vi "SO2 43c Serial Data Recording & DECADEv3.6.vi"() -> ()   [LabVIEW 2014]
uses:
  <vilib>/Instr/_visa.llb/VISA Set IO Buffer Mask.ctl
  <vilib>/Platform/TimedLoop/XDataNode/timing_clust.ctl
  <vilib>/Platform/TimedLoop/XDataNode/nitl_modes.ctl
  <vilib>/Platform/TimedLoop/XDataNode/wakeup.ctl
  C:/Program Files (x86)/National Instruments/LabVIEW 2014/examples/Data Communication/Network Streams/Simple Network Streams/support/Network Stream Command.ctl
  <vilib>/Utility/error.llb/whitespace.ctl
  <vilib>/Instr/_visa.llb/VISA Configure Serial Port (Instr).vi
  <vilib>/Utility/tcp.llb/UDP Multicast Write-Only Open.vi
  <vilib>/platform/TimedLoop/XDataNode/XDataNode.xnode
  <vilib>/Platform/TimedLoop/XDataNode/XDNodeRunTimeDep.lvlib
panel:
  out "Default file name":string
  out "Stop File Write":bool
  out "error out 4":errorcluster
  out "Data Array UDP":string[](array[string])
  out "Slope":dbl=0.87463
  out "Offset":dbl
  out "Simulate TWA Conc":dbl
  out "8hr_TWA_limit":i32=490
  out "10mins_STEL_limit":i32=700
  out "Simulate STEL Conc":dbl
  out "Simulate\nconc":bool
  out "q_size 2":i32
  out "8hr_so2_avg 2":dbl=1.0
  out "10min_so2_avg":dbl=1.0
  out "q_size":i32
  in  "Clear Display\nErrors":bool
  in  "dummy2":string="0"
  out "Data Processing":bool
  out "Serial Visa Error":errorcluster
  out "SEPTIC TCP Error Out":errorcluster
  out "TCP packet\nSend to SEPTIC":bool
  in  "Time Stamp\nOffset":u32=1
  out "Data Array TCP":string[](array[string])
  out "UDP packet \nstatus":bool
  out "UDP_Out_Error":errorcluster
  out "FISH TCP Error Out":errorcluster
  out "TCP packet\nSend to FISH":bool
  out "TCP Binary Packet":string
  out "Scan from String Error Counter\nfrom process loop":i32
  out "Read Error Counter\nfrom process loop":i32
  in  "milliseconds to wait":u32=330
  in  "ID":string="«"
  in  "VISA resource name":refnum<visa-resource-name>="ASRL6::INSTR"
  out "Data In Array":string[](array[string])
  out "UDP_ASCII_Out":string
  out "UDP_Pack_num":u32
  out "Flight Number":string
  in  "dummy1":string="00"
  out "Data String":string
  out "Internal packet":string[](array[string])
  out "RAW DATA":string
  in  "stop":bool
  out "Number of Send & Read Error\nfrom Acquire Loop":i32
  out "Command In":string
  # "SO2_conc"
  # "PMT_Volt"
  # "Lamp_Volt"
  # "Lamp_Intensity_Hz"
  # "Internal_Temp_degC"
  # "Reaction_Chamber_Temp_degC"
  # "Reaction_Chamber_Press_mmHg"
  # "Sample_Flow_litre_per_minute"
  # "Flag"
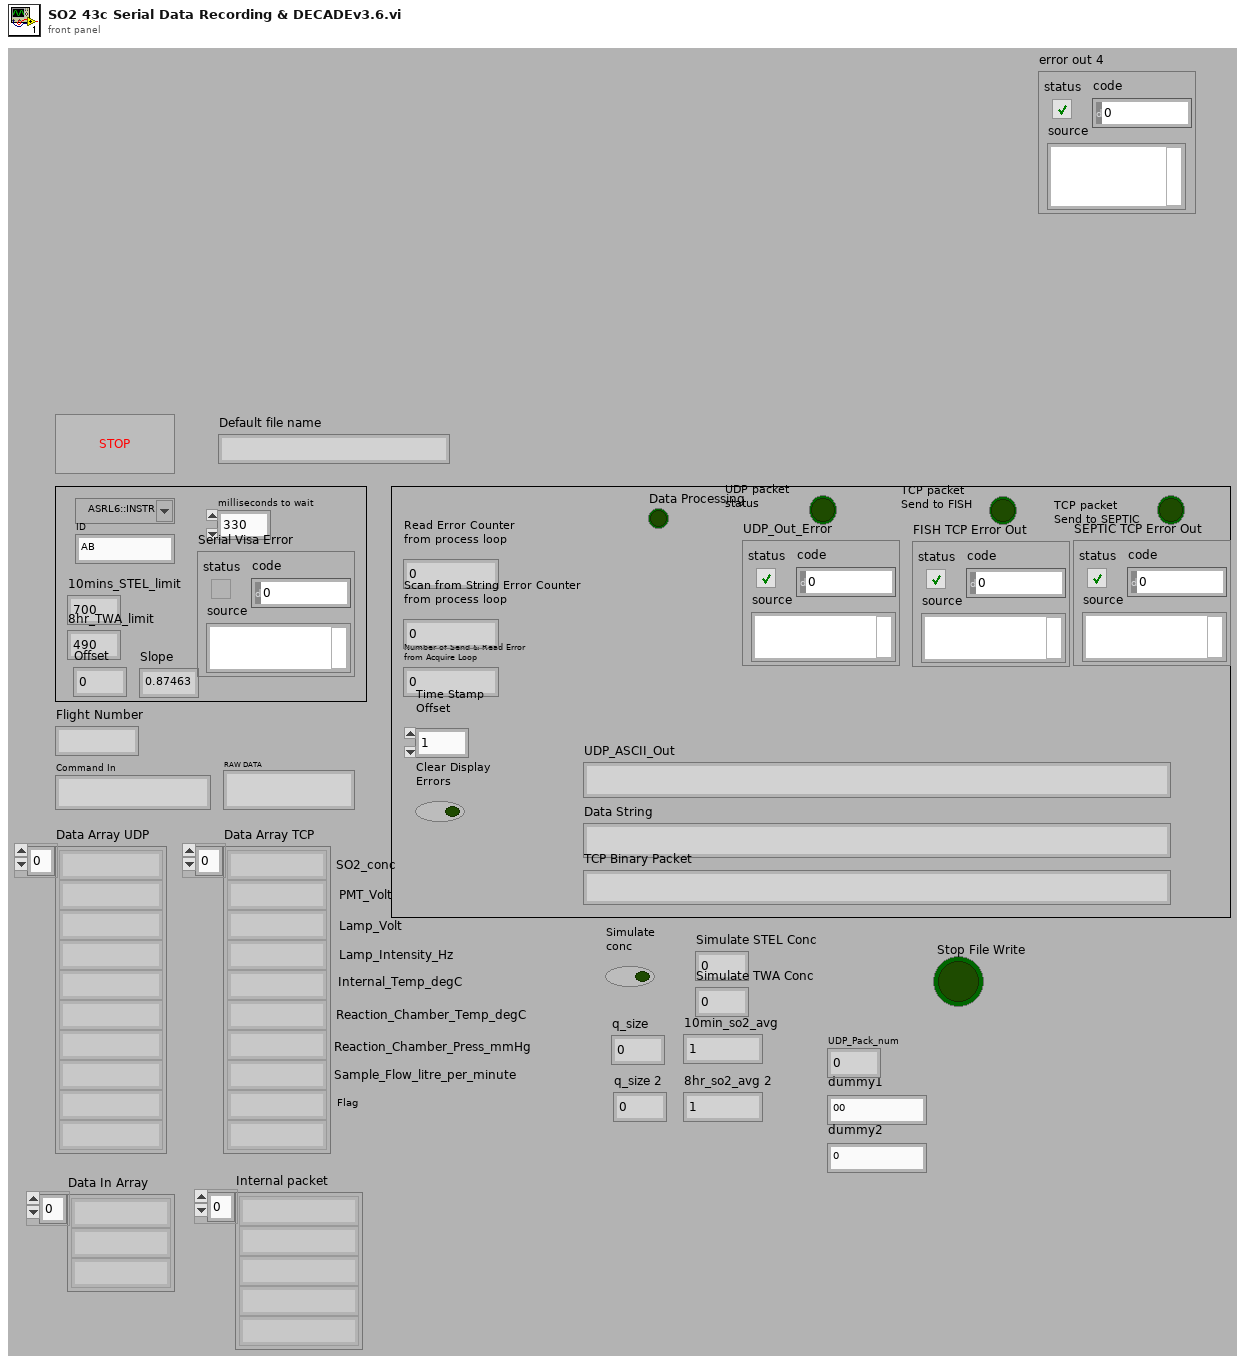
[diagram p1: front panel]
types:
  T1 = typedef "VISA Set IO Buffer Mask.ctl" = u16
  T2 = typedef "Network Stream Command.ctl" = cluster{"Message":string, "Message Data":variant}
  T3 = typedef "XDNodeRunTimeDep.lvlib/timing_clust.ctl" = cluster{"Expected End [f-1]":u64, "Actual End [f-1]":u64, "Finished Late? [f-1]":bool, "Expected End [i-1]":u64, "Actual End [i-1]":u64, "Finished Late? [i-1]":bool, "Expected Start [i]":u64, "Actual Start [i]":u64, "Expected Start [f]":u64, "Actual Start [f]":u64, "Source Name":string, "Structure Name":string, "Period":i64, "Deadline":i64, "Offset":i64, "Start":i64, "Priority":i32, "Timeout":i32, "Mode":T4, "Wakeup Reason":T5, "Error":errorcluster, "Source Type":string, "Secondary Source Type":string, "Global End Time":u64, "Global Start Time":u64, "Frame Duration":u64, "Iteration Duration":u64, "Assigned CPU":i32, "I/O Scan Engine Mode":u32}
  T4 = typedef "XDNodeRunTimeDep.lvlib/nitl_modes.ctl" = enum32{"No Change", "Process missed periods, maintain original phase", "Discard missed periods, maintain original phase", "Process missed periods, ignore original phase", "Discard missed periods, ignore original phase"}
  T5 = typedef "XDNodeRunTimeDep.lvlib/wakeup.ctl" = enum32{"Normal", "Aborted", "Asynchronous wakeup", "Timing source error", "Timed loop error", "Timeout"}
  T6 = enum16{"open", "replace", "create", "open or create", "replace or create", "replace or create with confirmation"}
  T7 = typedef "whitespace.ctl" = u16
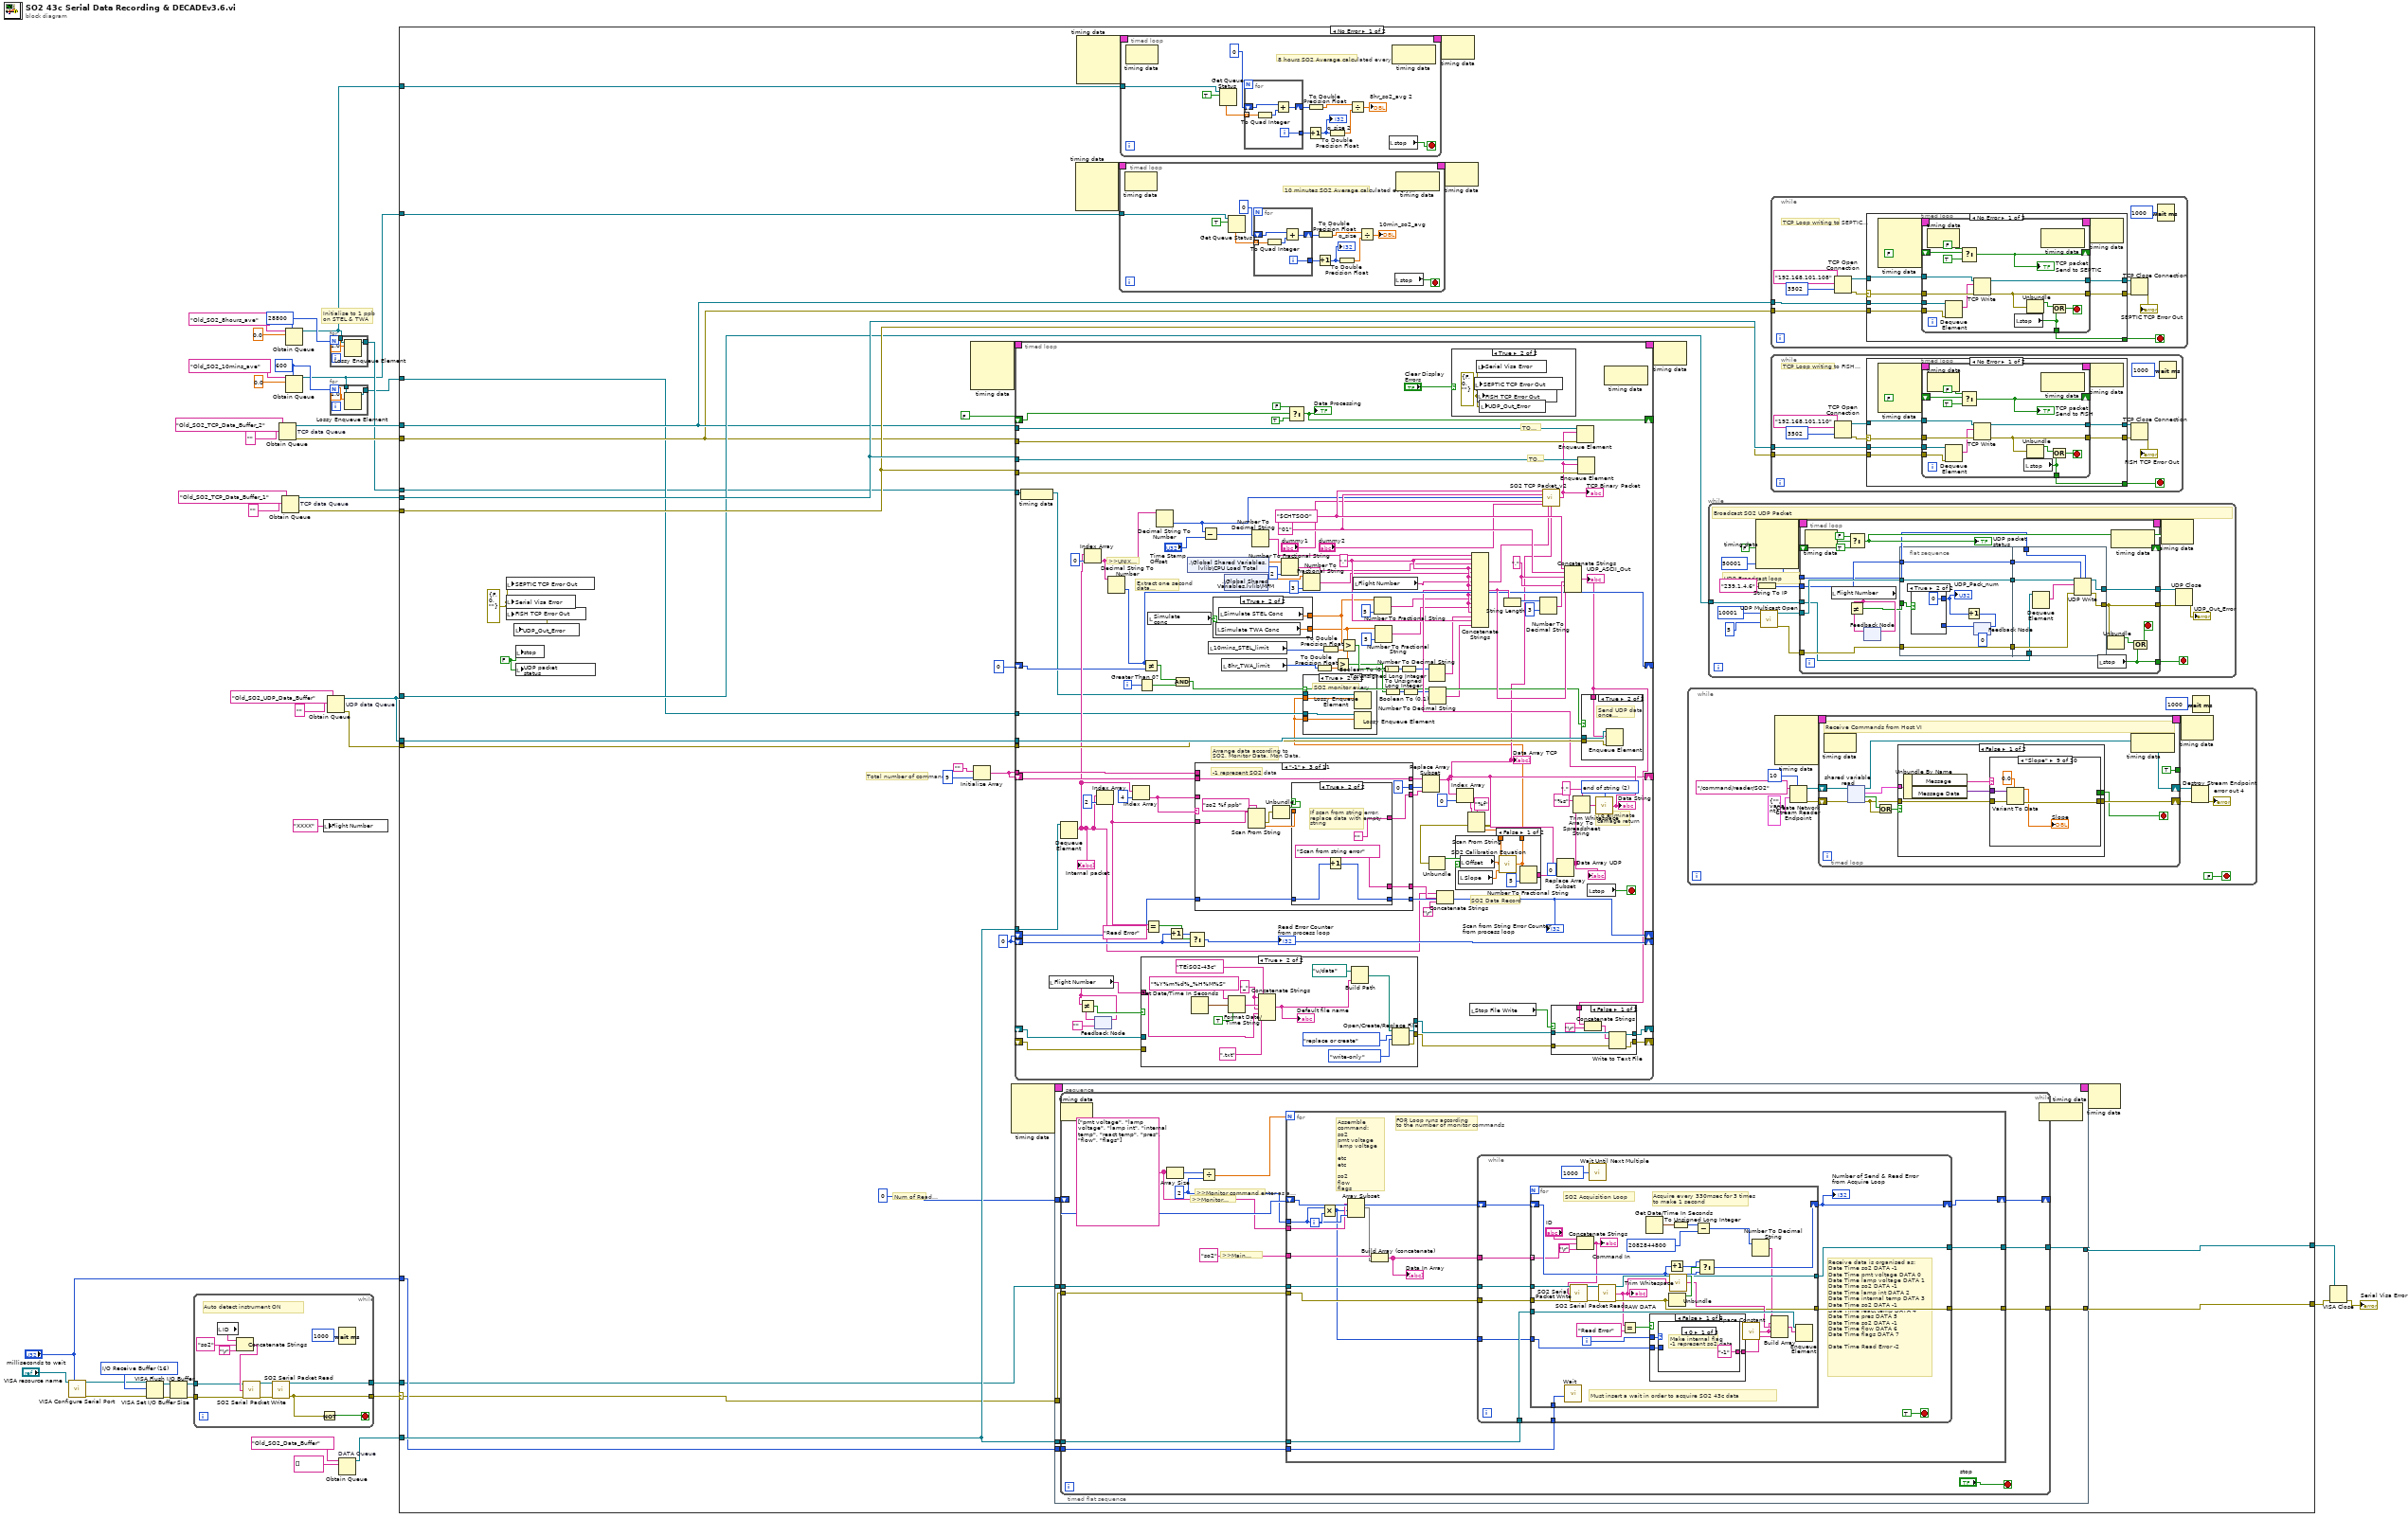
[diagram p0: block diagram]
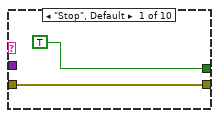
[diagram p2: hidden frame]
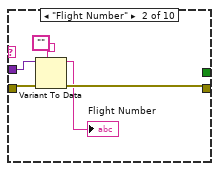
[diagram p3: hidden frame]
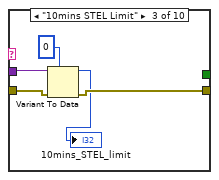
[diagram p4: hidden frame]
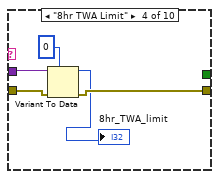
[diagram p5: hidden frame]
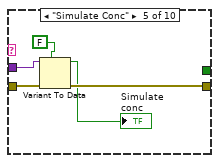
[diagram p6: hidden frame]
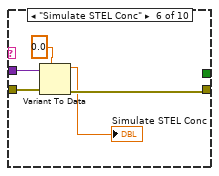
[diagram p7: hidden frame]
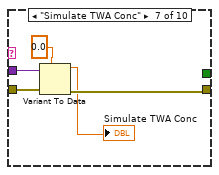
[diagram p8: hidden frame]
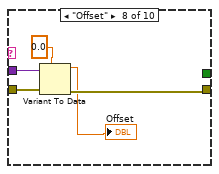
[diagram p9: hidden frame]
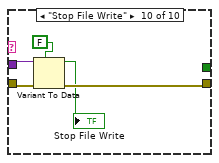
[diagram p10: hidden frame]
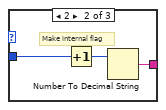
[diagram p12: hidden frame]
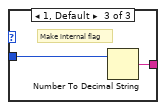
[diagram p13: hidden frame]
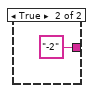
[diagram p14: hidden frame]
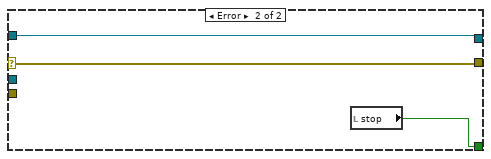
[diagram p15: hidden frame]
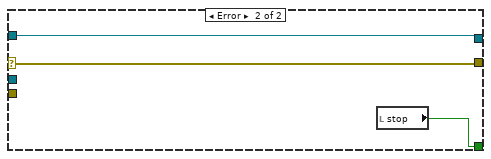
[diagram p17: hidden frame]
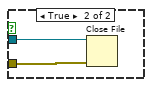
[diagram p19: hidden frame]
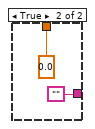
[diagram p20: hidden frame]
diagram:
  w10 = T1 16 items=["I/O Receive Buffer"=16, "I/O Transmit Buffer"=32, "I/O Receive and Transmit Buffer"=48] ("Mask")
  w16 = 28800 ("max queue size (-1, unlimited)")
  w13 = 600 ("max queue size (-1, unlimited)")
  # "Initialise to 1 ppb\non STEL & TWA"
  n1 = call-poly "VISA Configure Serial Port"("VISA resource name"="VISA resource name", "timeout (10sec)"="milliseconds to wait") -> ("VISA resource name out"=w9:refnum<visa-resource-name>, "error out"=w8:errorcluster)  [unwired: 12 in]
  n2 = VISA Set I/O Buffer Size(VISA resource name=w9, mask (16)=w10, error in (no error)=w8) -> (VISA resource name out=w6:refnum<visa-resource-name>, error out=w7:errorcluster)  [unwired: 1 in]
  n3 = VISA Flush I/O Buffer(VISA resource name=w6, error in (no error)=w7) -> (VISA resource name out=w5:refnum<visa-resource-name>, error out=w4:errorcluster)  [unwired: 1 in]
  n4 = while {
    tunnel: w5 -> [w48]
    tunnel: w4 -> [w47]
    tunnel: [w43] -> w3
    tunnel: [w42] -> w2
    stop <- w44 stop-if-true
    # "Auto detect instrument ON"
    n5 = local read "ID"() -> (w51:string)
    n6 = Concatenate Strings(w51, "so2" ("string"), "\r") -> (w49:string)
    n7 = call "SO2 Serial Packet Write.vi"("VISA resource name In"=w48, "Data in"=w49, "error in (no error)"=w47) -> ("VISA resource name Out"=w45:refnum<visa-resource-name>, "error out"=w46:errorcluster)  [unwired: 11 in]
    n8 = call "SO2 Serial Packet Read.vi"("VISA resource In"=w45, "error in"=w46) -> ("VISA resource Out"=w42:refnum<visa-resource-name>, "error out"=w43:errorcluster)  [unwired: 11 in, 1 out]
    n9 = Not(x=w43) -> (.not. x?=w44:bool)
    n10 = Wait (ms)(milliseconds to wait=u32 1000) -> ()  [unwired: 1 out]
  }
  n11 = Obtain Queue "TCP data Queue"(name (unnamed)="Old_SO2_TCP_Data_Buffer_2", element data type="") -> (queue out=w23:refnum<queue>, error out=w22:errorcluster)  [unwired: 3 in, 1 out]
  n12 = Obtain Queue "TCP data Queue"(name (unnamed)="Old_SO2_TCP_Data_Buffer_1", element data type="") -> (queue out=w31:refnum<queue>, error out=w30:errorcluster)  [unwired: 3 in, 1 out]
  n13 = Obtain Queue(max queue size (-1, unlimited)=w16, name (unnamed)="Old_SO2_8hours_ave", element data type=0.0 ("index")) -> (queue out=w15:refnum<queue>)  [unwired: 2 in, 2 out]
  n14 = Obtain Queue(max queue size (-1, unlimited)=w13, name (unnamed)="Old_SO2_10mins_ave", element data type=0.0 ("index")) -> (queue out=w12:refnum<queue>)  [unwired: 2 in, 2 out]
  n15 = local write "Flight Number"("XXXX" ("Flight Number")) -> ()
  n16 = Obtain Queue "UDP data Queue"(name (unnamed)="Old_SO2_UDP_Data_Buffer", element data type="") -> (queue out=w26:refnum<queue>, error out=w27:errorcluster)  [unwired: 3 in, 1 out]
  n17 = for {
    N: w16 -> [_]
    tunnel: w15 -> [w55]
    tunnel: [w54] -> w14
    n18 = Lossy Enqueue Element(queue=w55, element=1.0) -> (queue out=w54:refnum<queue>)  [unwired: 1 in, 3 out]
  }
  n19 = for {
    N: w13 -> [_]
    tunnel: [w58] -> w11
    tunnel: w12 -> [w56]
    n20 = Lossy Enqueue Element(queue=w56, element=1.0) -> (queue out=w58:refnum<queue>)  [unwired: 1 in, 3 out]
  }
  n21 = Obtain Queue "DATA Queue"(name (unnamed)="Old_SO2_Data_Buffer", element data type=string[] []) -> (queue out=w38:refnum<queue>)  [unwired: 3 in, 2 out]
  n22 = case shown="No Error" w3 {
    selector: w3 -> [w61 w818]
    tunnel: [w92 w818] -> w35
    tunnel: [w91 w817] -> w36
    tunnel: w38 -> [w88 _]
    tunnel: w2 -> [w62 w817]
    tunnel: w31 -> [w81 _]
    tunnel: w30 -> [w80 _]
    tunnel: w26 -> [w79 _]
    tunnel: w27 -> [w78 _]
    tunnel: w26 -> [w77 _]
    tunnel: w23 -> [w75 _]
    tunnel: w22 -> [w74 _]
    tunnel: "milliseconds to wait" -> [w73 _]
    tunnel: w12 -> [w70 _]
    tunnel: w15 -> [w69 _]
    tunnel: w11 -> [w68 _]
    tunnel: w14 -> [w67 _]
    frame No Error {
      w71 = errorcluster {"status"=FALSE, "code"=0, "source"=""} ("UDP Error Out")
      w83 = 0
      w82 = FALSE ("stop")
      # "Num of Read Error"
      # "Total number of commands"
      n23 = local write "SEPTIC TCP Error Out"(w71) -> ()
      n24 = local write "Serial Visa Error"(w71) -> ()
      n25 = local write "FISH TCP Error Out"(w71) -> ()
      n26 = local write "UDP_Out_Error"(w71) -> ()
      n27 = local write "stop"(w82) -> ()
      n28 = local write "UDP packet \nstatus"(w82) -> ()
      n29 = node-c288() -> (w90:T3)  [unwired: 4 in]
      n30 = Initialize Array("", 9) -> (w84:string[])
      n31 = node-c288() -> (w60:T3)  [unwired: 4 in]
      n32 = timed-loop {
        timing: w90 -> [_]
        timing-out: [_] -> w89
        tunnel: w88 -> [w564]
        shift-right: [w481] -> _
        shift-left: w84 -> [w554]
        shift-right: [w545] -> _
        shift-left: w83 -> [w542]
        tunnel: w84 -> [w544]
        shift-right: [w540] -> _
        shift-left: w83 -> [w541]
        tunnel: w81 -> [w535]
        tunnel: w80 -> [w534]
        tunnel: w79 -> [w533]
        tunnel: w78 -> [w532]
        shift-right: [w524] -> _
        shift-left: 0 -> [w527]
        tunnel: w75 -> [w523]
        tunnel: w74 -> [w522]
        shift-right: [w513] -> _
        shift-left: FALSE -> [w516]
        tunnel: w68 -> [w507]
        tunnel: w67 -> [w506]
        shift-right: [w466] -> _
        shift-left: _ -> [w463]
        shift-right: [w465] -> _
        shift-left: _ -> [w461]
        i -> [w525]
        stop <- w562 stop-if-true
        w550 = T7 2 items=["both", "start of string", "end of string"] ("location (both)")
        w505 = ","
        w537 = "01"
        w556 = ","
        w538 = "$CHTSOO"
        # "TO SEPTIC"
        # "TO FISH"
        # "Extract one second data\nfor UDP sending"
        # "Arrange data according to\nSO2, Monitor Data, Mon Data,"
        # "To eliminate\ncarriage return"
        # ">>UNIX TIME>>"
        # "SO2 Data Record"
        n33 = node-c288() -> ()  [unwired: 1 in]
        n34 = local read "Flight Number"() -> (w462:string)
        n35 = Dequeue Element(queue=w564) -> (element=w530:string[])  [unwired: 2 in, 3 out]
        "Internal packet" <- w530
        n36 = Index Array(array=w530, index=0) -> (element=w529:string)
        n37 = feedback #1("" ("Flight Number")) -> (w471:string)
        n38 = Not Equal?(x=w462, y=w471) -> (x != y?=w469:bool)
        n39 = feedback-in #1(w462) -> ()
        n40 = Index Array(array=w530, index=2) -> (element=w548:string)
        n41 = Decimal String To Number(string=w529) -> (number=w524:i32)  [unwired: 2 in, 1 out]
        n42 = Index Array(array=w530, index=4) -> (element=w512:string)
        n43 = Greater Than 0?(x=w525) -> (x > 0?=w528:bool)
        n44 = case shown="True" w469 {
          tunnel: [w566 w569] -> w468
          tunnel: [w565 w568] -> w464
          tunnel: w463 -> [w566 _]
          tunnel: w461 -> [w565 _]
          tunnel: w462 -> [_ w567]
          frame False {
          }
          frame True {
            w576 = "_" ("string")
            n45 = Get Date/Time In Seconds() -> (seconds since 1Jan1904=w577:timestamp)
            n46 = Format Date/Time String(time format string (%c)="%Y%m%d%_%H%M%S", seconds (now)=w577, UTC format=TRUE) -> (date/time string=w580:string)
            n47 = Concatenate Strings("TEiSO2-43c" ("string"), w576, w580, w576, w567, ".txt" ("string")) -> (w574:string)
            "Default file name" <- w574
            n48 = Build Path(base path=path "u:/data", name or relative path=w574) -> (appended path=w570:path)
            n49 = Open/Create/Replace File(file path (use dialog)=w570, operation (0:open)=T6."replace or create", access (0:read/write)=enum16{"read/write", "read-only", "write-only"}."write-only") -> (refnum out=w569:refnum<file>, error out=w568:errorcluster)  [unwired: 3 in, 1 out]
          }
        }
        n50 = Not Equal?(x=w524, y=w527) -> (x != y?=w526:bool)
        n51 = Equal?(x=w548, y="Read Error") -> (x = y?=w546:bool)
        n52 = local read "Simulate\nconc"() -> (w475:bool)
        n53 = Decimal String To Number(string=w529) -> (number=w519:i32)  [unwired: 2 in, 1 out]
        n54 = Increment(x=w542) -> (x+1=w543:i32)
        n55 = Compound Arithmetic op=AND(w526, w528) -> (w508:bool)
        n56 = shared-variable ".\\Global Shared Variables.lvlib\\CPU Load Total"() -> (w459:dbl)  [unwired: 1 in, 1 out]
        n57 = Select(t=w543, s=w546, f=w542) -> (s? t:f=w545:i32)
        "Read Error Counter\nfrom process loop" <- w545
        n58 = case shown="\"-1\"" w512 {
          tunnel: w512 -> [w616 _ _ w652 w673 w694 w716 w738 w760 w782 w804]
          tunnel: w554 -> [w617 _ w631 w653 w674 w695 w717 w739 w761 w783 w805]
          tunnel: w548 -> [_ _ w628 w648 w669 w691 w713 w735 w757 w779 w801]
          tunnel: [w617 w620 w631 w653 w674 w695 w717 w739 w761 w783 w805] -> w488
          tunnel: [w614 _ 0 ("index") w650 w671 w692 w714 w736 w758 w780 w802] -> w487
          tunnel: [_ _ w627 w647 w668 w690 w712 w734 w756 w778 w796] -> w553
          tunnel: w544 -> [_ w620 _ _ _ _ _ _ _ _ _]
          tunnel: w541 -> [w612 w619 w624 w644 w665 w685 w708 w729 w752 w773 w795]
          tunnel: [w612 w619 w623 w643 w664 w684 w707 w728 w751 w772 w794] -> w540
          tunnel: ["Internal False Flag Detected" "" w622 w642 w663 w683 w706 w727 w750 w771 w793] -> w539
          frame "False", Default {
            n59 = Decimal String To Number(string=w616) -> (number=w613:i32)  [unwired: 2 in, 1 out]
            n60 = Add(x=w613, y=1) -> (x+y=w614:i32)
          }
          frame "-2" {
            # "Read Error Detected\nMake all data as a space"
          }
          frame "-1" {
            # "-1 represent SO2 data"
            n61 = Scan From String(format string="so2 %f ppb", input string=w628) -> (error out=w626:errorcluster, output 1=w621:dbl)  [unwired: 3 in, 2 out]
            n62 = Unbundle(w626) -> ("status"=w625:bool)  [unwired: 2 out]
            n63 = case shown="True" w625 {
              tunnel: w621 -> [w632 _]
              tunnel: [w636 ""] -> w627
              tunnel: w624 -> [w635 w640]
              tunnel: [w635 w639] -> w623
              tunnel: ["" "Scan from string error"] -> w622
              frame False {
                # "Extract the concentration\nvalue & fixed format"
                n64 = Number To Fractional String(number=w632, precision (6)=i16 5) -> (F-format string=w636:string)  [unwired: 2 in]
              }
              frame True {
                # "If scan from string error,\nreplace data with empty\nstring"
                n65 = Increment(x=w640) -> (x+1=w639:i32)
              }
            }
          }
          frame "0" {
            # "0 represents pmt voltage -0510 volts"
            n66 = Scan From String(format string="pmt voltage %d volts", input string=w648) -> (error out=w646:errorcluster, output 1=w641:i32)  [unwired: 3 in, 2 out]
            n67 = Decimal String To Number(string=w652) -> (number=w651:i32)  [unwired: 2 in, 1 out]
            n68 = Unbundle(w646) -> ("status"=w645:bool)  [unwired: 2 out]
            n69 = case shown="False" w645 {
              tunnel: w641 -> [w657 _]
              tunnel: [w654 w658] -> w647
              tunnel: w644 -> [w656 w661]
              tunnel: [w656 w660] -> w643
              tunnel: ["" "Scan from string error"] -> w642
              tunnel: [w654 w658] -> _
              frame False {
                # "Extract the actual value\n& fixed format"
                n70 = Number To Decimal String(number=w657) -> (decimal integer string=w654:string)  [unwired: 1 in]
              }
              frame True {
                w658 = ""
                # "If scan from string error,\nreplace data with empty\nstring"
                n71 = Increment(x=w661) -> (x+1=w660:i32)
              }
            }
            n72 = Increment(x=w651) -> (x+1=w650:i32)
          }
          frame "1" {
            # "1 represents lamp voltage; lamp voltage 810 volts"
            n73 = Scan From String(format string="lamp voltage %d volts", input string=w669) -> (error out=w667:errorcluster, output 1=w662:i32)  [unwired: 3 in, 2 out]
            n74 = Decimal String To Number(string=w673) -> (number=w672:i32)  [unwired: 2 in, 1 out]
            n75 = Unbundle(w667) -> ("status"=w666:bool)  [unwired: 2 out]
            n76 = case shown="True" w666 {
              tunnel: w662 -> [w678 _]
              tunnel: [w675 w679] -> w668
              tunnel: w665 -> [w677 w682]
              tunnel: [w677 w681] -> w664
              tunnel: ["" "Scan from string error"] -> w663
              tunnel: [w675 w679] -> _
              frame False {
                # "Extract the actual value\n& fixed format"
                n77 = Number To Decimal String(number=w678) -> (decimal integer string=w675:string)  [unwired: 1 in]
              }
              frame True {
                w679 = ""
                # "If scan from string error,\nreplace data with empty\nstring"
                n78 = Increment(x=w682) -> (x+1=w681:i32)
              }
            }
            n79 = Increment(x=w672) -> (x+1=w671:i32)
          }
          frame "2" {
            # "2 represents lamp intensity; lamp int 35867 Hz"
            n80 = Scan From String(format string="lamp int %d Hz", input string=w691) -> (error out=w687:errorcluster, output 1=w688:i32)  [unwired: 3 in, 2 out]
            n81 = Decimal String To Number(string=w694) -> (number=w693:i32)  [unwired: 2 in, 1 out]
            n82 = Unbundle(w687) -> ("status"=w686:bool)  [unwired: 2 out]
            n83 = case shown="True" w686 {
              tunnel: [w696 w701] -> w690
              tunnel: w688 -> [w700 _]
              tunnel: w685 -> [w699 w704]
              tunnel: [w699 w703] -> w684
              tunnel: ["" "Scan from string error"] -> w683
              tunnel: [w696 w701] -> _
              frame False {
                # "Extract the actual value\n& fixed format"
                n84 = Number To Fractional String(number=w700, precision (6)=i16 0) -> (F-format string=w696:string)  [unwired: 2 in]
              }
              frame True {
                w701 = ""
                # "If scan from string error,\nreplace data with empty\nstring"
                n85 = Increment(x=w704) -> (x+1=w703:i32)
              }
            }
            n86 = Increment(x=w693) -> (x+1=w692:i32)
          }
          frame "3" {
            # "3 represents internal temp; internal temp 027.2 deg C, actual 027.2"
            n87 = Scan From String(format string="%[^,], %s %f", input string=w713) -> (error out=w710:errorcluster, output 3=w705:dbl)  [unwired: 7 in, 2 out]
            n88 = Decimal String To Number(string=w716) -> (number=w715:i32)  [unwired: 2 in, 1 out]
            n89 = Unbundle(w710) -> ("status"=w709:bool)  [unwired: 2 out]
            n90 = case shown="True" w709 {
              tunnel: [w718 w723] -> w712
              tunnel: w705 -> [w722 _]
              tunnel: w708 -> [w721 w726]
              tunnel: [w721 w725] -> w707
              tunnel: ["" "Scan from string error"] -> w706
              tunnel: [w718 w723] -> _
              frame False {
                # "Extract the actual value\n& fixed format"
                n91 = Number To Fractional String(number=w722, precision (6)=i16 1) -> (F-format string=w718:string)  [unwired: 2 in]
              }
              frame True {
                w723 = ""
                # "If scan from string error,\nreplace data with empty\nstring"
                n92 = Increment(x=w726) -> (x+1=w725:i32)
              }
            }
            n93 = Increment(x=w715) -> (x+1=w714:i32)
          }
          frame "4" {
            # "4 represents react temp; react temp 045.2 deg C"
            n94 = Scan From String(format string="react temp %f deg C", input string=w735) -> (error out=w731:errorcluster, output 1=w732:dbl)  [unwired: 3 in, 2 out]
            n95 = Decimal String To Number(string=w738) -> (number=w737:i32)  [unwired: 2 in, 1 out]
            n96 = Unbundle(w731) -> ("status"=w730:bool)  [unwired: 2 out]
            n97 = case shown="False" w730 {
              tunnel: [w740 w745] -> w734
              tunnel: w732 -> [w744 _]
              tunnel: w729 -> [w743 w748]
              tunnel: [w743 w747] -> w728
              tunnel: ["" "Scan from string error"] -> w727
              tunnel: [w740 w745] -> _
              frame False {
                # "Extract the actual value\n& fixed format"
                n98 = Number To Fractional String(number=w744, precision (6)=i16 1) -> (F-format string=w740:string)  [unwired: 2 in]
              }
              frame True {
                w745 = ""
                # "If scan from string error,\nreplace data with empty\nstring"
                n99 = Increment(x=w748) -> (x+1=w747:i32)
              }
            }
            n100 = Increment(x=w737) -> (x+1=w736:i32)
          }
          frame "5" {
            # "5 represents chamber pressure; pres 760.0 mm Hg, actual 753.4"
            n101 = Scan From String(format string="%[^,], %s %f", input string=w757) -> (error out=w754:errorcluster, output 3=w749:dbl)  [unwired: 7 in, 2 out]
            n102 = Decimal String To Number(string=w760) -> (number=w759:i32)  [unwired: 2 in, 1 out]
            n103 = Unbundle(w754) -> ("status"=w753:bool)  [unwired: 2 out]
            n104 = case shown="False" w753 {
              tunnel: [w762 w767] -> w756
              tunnel: w749 -> [w766 _]
              tunnel: w752 -> [w765 w770]
              tunnel: [w765 w769] -> w751
              tunnel: ["" "Scan from string error"] -> w750
              tunnel: [w762 w767] -> _
              frame False {
                # "Extract the actual value\n& fixed format"
                n105 = Number To Fractional String(number=w766, precision (6)=i16 1) -> (F-format string=w762:string)  [unwired: 2 in]
              }
              frame True {
                w767 = ""
                # "If scan from string error,\nreplace data with empty\nstring"
                n106 = Increment(x=w770) -> (x+1=w769:i32)
              }
            }
            n107 = Increment(x=w759) -> (x+1=w758:i32)
          }
          frame "6" {
            # "6 represents flow data; flow 0.503 l/m"
            n108 = Scan From String(format string="flow %f l/m", input string=w779) -> (error out=w775:errorcluster, output 1=w776:dbl)  [unwired: 3 in, 2 out]
            n109 = Decimal String To Number(string=w782) -> (number=w781:i32)  [unwired: 2 in, 1 out]
            n110 = Unbundle(w775) -> ("status"=w774:bool)  [unwired: 2 out]
            n111 = case shown="True" w774 {
              tunnel: [w788 ""] -> w778
              tunnel: w776 -> [w787 _]
              tunnel: w773 -> [w786 w791]
              tunnel: [w786 w790] -> w772
              tunnel: ["" "Scan from string error"] -> w771
              frame False {
                # "Extract the actual value\n& fixed format"
                n112 = Number To Fractional String(number=w787, precision (6)=i16 3) -> (F-format string=w788:string)  [unwired: 2 in]
              }
              frame True {
                # "If scan from string error,\nreplace data with empty\nstring"
                n113 = Increment(x=w791) -> (x+1=w790:i32)
              }
            }
            n114 = Increment(x=w781) -> (x+1=w780:i32)
          }
          frame "7" {
            # "7 represents flags data; flags 1c100000"
            n115 = Scan From String(format string="flags %s", input string=w801) -> (error out=w799:errorcluster, output 1=w797:string)  [unwired: 3 in, 2 out]
            n116 = Decimal String To Number(string=w804) -> (number=w803:i32)  [unwired: 2 in, 1 out]
            n117 = Unbundle(w799) -> ("status"=w798:bool)  [unwired: 2 out]
            n118 = case shown="False" w798 {
              tunnel: w797 -> [w808 _]
              tunnel: [w808 ""] -> w796
              tunnel: w795 -> [w807 w811]
              tunnel: [w807 w810] -> w794
              tunnel: ["" "Scan from string error"] -> w793
              frame False {
                # "Extract the actual value\n& fixed format"
              }
              frame True {
                # "If scan from string error,\nreplace data with empty\nstring"
                n119 = Increment(x=w811) -> (x+1=w810:i32)
              }
            }
            n120 = Increment(x=w803) -> (x+1=w802:i32)
          }
        }
        "Scan from String Error Counter\nfrom process loop" <- w540
        n121 = Subtract(x=w519, y="Time Stamp\nOffset") -> (x-y=w520:u32)
        n122 = local read "10mins_STEL_limit"() -> (w473:i32)
        n123 = case shown="True" w475 {
          tunnel: [w600 w602] -> w501
          tunnel: [w599 w601] -> w499
          frame False {
            n124 = local read "10min_so2_avg"() -> (w600:dbl)
            n125 = local read "8hr_so2_avg 2"() -> (w599:dbl)
          }
          frame True {
            n126 = local read "Simulate TWA Conc"() -> (w601:dbl)
            n127 = local read "Simulate STEL Conc"() -> (w602:dbl)
          }
        }
        n128 = local read "8hr_TWA_limit"() -> (w472:i32)
        n129 = shared-variable ".\\Global Shared Variables.lvlib\\MFM"() -> (w457:dbl)  [unwired: 1 in, 1 out]
        n130 = Number To Decimal String(number=w520) -> (decimal integer string=w517:string)  [unwired: 1 in]
        n131 = Number To Fractional String(number=w459, precision (6)=i16 2) -> (F-format string=w455:string)  [unwired: 2 in]
        n132 = Select(t=FALSE, s=w516, f=TRUE) -> (s? t:f=w513:bool)
        "Data Processing" <- w513
        n133 = Number To Fractional String(number=w457, precision (6)=i16 3) -> (F-format string=w454:string)  [unwired: 2 in]
        n134 = To Double Precision Float(number=w472) -> (double precision float=w502:dbl)
        n135 = To Double Precision Float(number=w473) -> (double precision float=w503:dbl)
        n136 = Greater?(x=w499, y=w502) -> (0:w492:bool)
        n137 = Greater?(x=w501, y=w503) -> (0:w494:bool)
        n138 = local read "Flight Number"() -> (w474:string)
        n139 = Number To Fractional String(number=w501, precision (6)=i16 5) -> (F-format string=w498:string)  [unwired: 2 in]
        n140 = Number To Fractional String(number=w499, precision (6)=i16 5) -> (F-format string=w497:string)  [unwired: 2 in]
        n141 = Boolean To (0,1)(Boolean=w494) -> (0, 1=w496:i16)
        n142 = Boolean To (0,1)(Boolean=w492) -> (0, 1=w495:i16)
        n143 = To Unsigned Long Integer(number=w496) -> (unsigned 32bit integer=w490:u32)
        n144 = To Unsigned Long Integer(number=w495) -> (unsigned 32bit integer=w489:u32)
        n145 = Replace Array Subset(array=w488, new element=w553, index=w487) -> (w481:string[])
        "Data Array TCP" <- w481
        n146 = Number To Decimal String(number=w490) -> (decimal integer string=w493:string)  [unwired: 1 in]
        n147 = Number To Decimal String(number=w489) -> (decimal integer string=w491:string)  [unwired: 1 in]
        n148 = Concatenate Strings(w530, w539, "\r") -> ()  [unwired: 1 out]
        n149 = case shown="True" "Clear Display\nErrors" {
          frame False {
          }
          frame True {
            w607 = errorcluster {"status"=FALSE, "code"=0, "source"=""} ("UDP Error Out")
            n150 = local write "SEPTIC TCP Error Out"(w607) -> ()
            n151 = local write "Serial Visa Error"(w607) -> ()
            n152 = local write "FISH TCP Error Out"(w607) -> ()
            n153 = local write "UDP_Out_Error"(w607) -> ()
          }
        }
        n154 = Index Array(array=w481, index=0) -> (element=w485:string)
        n155 = Scan From String(format string="%f", input string=w485) -> (error out=w477:errorcluster, output 1=w483:dbl)  [unwired: 3 in, 2 out]
        n156 = Unbundle(w477) -> ("status"=w476:bool)  [unwired: 2 out]
        n157 = case shown="False" w476 {
          tunnel: w483 -> [w595 _]
          tunnel: [w594 ""] -> w482
          tunnel: [w593 0.0 ("Output")] -> w478
          frame False {
            n158 = local read "Slope"() -> (w591:dbl)
            n159 = local read "Offset"() -> (w592:dbl)
            n160 = call "SO2 Calibration Equation.vi"("Input"=w595, "Offset"=w592, "Slope"=w591) -> ("Output"=w593:dbl)  [unwired: 12 in]
            n161 = Number To Fractional String(number=w593, precision (6)=i16 5) -> (F-format string=w594:string)  [unwired: 2 in]
          }
          frame True {
          }
        }
        n162 = case shown="True" w508 {
          tunnel: w507 -> [_ w606]
          tunnel: w478 -> [_ w603]
          tunnel: w478 -> [_ w605]
          tunnel: w506 -> [_ w604]
          frame False {
          }
          frame True {
            # "SO2 monitor every second"
            n163 = Lossy Enqueue Element(queue=w606, element=w603) -> ()  [unwired: 1 in, 4 out]
            n164 = Lossy Enqueue Element(queue=w604, element=w605) -> ()  [unwired: 1 in, 4 out]
          }
        }
        n165 = local read "Stop File Write"() -> (w467:bool)
        n166 = call "SO2 TCP Packet_v2.vi"("ID"=w538, "Version"=w537, "utc_time"=w519, "dummy1"="dummy1", "dummy2"="dummy2", "Flight Number"=w474, "Data Array"=w481) -> ("TCP Binary Packet"=w521:string)  [unwired: 8 in]
        "TCP Binary Packet" <- w521
        n167 = Replace Array Subset(array=w481, new element=w482, index=0) -> (w480:string[])
        "Data Array UDP" <- w480
        n168 = Array To Spreadsheet String(delimiter (Tab)=",", array=w480, 3:"%s" ("format string")) -> (spreadsheet string=w549:string)
        n169 = Enqueue Element(queue=w523, element=w521, error in (no error)=w522) -> ()  [unwired: 1 in, 3 out]
        n170 = Enqueue Element(queue=w535, element=w521, error in (no error)=w534) -> ()  [unwired: 1 in, 3 out]
        n171 = local read "stop"() -> (w562:bool)
        n172 = call <vilib>:"Trim Whitespace.vi"("string"=w549, "location (both)"=w550) -> ("trimmed string"=w511:string)
        "Data String" <- w511
        n173 = Concatenate Strings(w517, w505, w455, w505, w454, w505, w474, w505, w511, w505, w498, w505, w497, w505, w493, w505, w491) -> (w555:string)
        n174 = String Length(string=w555) -> (length=w559:i32)
        n175 = Number To Decimal String(number=w559, width (-)=i16 3) -> (decimal integer string=w557:string)
        n176 = Concatenate Strings(w538, w537, w556, w557, w556, w555) -> (w460:string)
        "UDP_ASCII_Out" <- w460
        n177 = case shown="False" w467 {
          tunnel: w460 -> [w586 _]
          tunnel: w468 -> [w588 w590]
          tunnel: w464 -> [w587 w589]
          tunnel: [w583 _] -> w466
          tunnel: [w582 _] -> w465
          frame False {
            n178 = Concatenate Strings(w586, "\r") -> (w584:string)
            n179 = Write to Text File(file (use dialog)=w588, text=w584, error in=w587) -> (refnum out=w583:refnum<file>, error out=w582:errorcluster)  [unwired: 2 out]
          }
          frame True {
            n180 = Close File(refnum=w590, error in=w589) -> ()  [unwired: 2 out]
          }
        }
        n181 = case shown="True" w508 {
          tunnel: w533 -> [_ w610]
          tunnel: w532 -> [_ w609]
          tunnel: w460 -> [_ w608]
          frame False {
          }
          frame True {
            # "Send UDP data once\na second"
            n182 = Enqueue Element(queue=w610, element=w608, error in (no error)=w609) -> ()  [unwired: 1 in, 3 out]
          }
        }
        n183 = node-c288() -> ()  [unwired: 1 in, 1 out]
      }
      n184 = timed-sequence {
        timing: w60 -> [_]
        timing-out: [_] -> w59
        tunnel: [w180] -> w92
        tunnel: [w179] -> w91
        tunnel: w88 -> [w178]
        tunnel: 0 -> [w177]
        tunnel: w73 -> [w176]
        tunnel: w62 -> [w175]
        tunnel: w61 -> [w174]
        n185 = timed-flat-sequence {
          tunnel: [w187] -> w180
          tunnel: [w186] -> w179
          tunnel: w178 -> [w185]
          tunnel: w177 -> [w184]
          tunnel: w176 -> [w183]
          tunnel: w175 -> [w182]
          tunnel: w174 -> [w181]
          n186 = node-c288() -> ()  [unwired: 1 in, 1 out]
          n187 = while {
            tunnel: [w190] -> w187
            tunnel: w182 -> [w201]
            tunnel: w181 -> [w200]
            tunnel: [w199] -> w186
            tunnel: w185 -> [w198]
            shift-right: [w196] -> _
            shift-left: w184 -> [w197]
            tunnel: w183 -> [w188]
            stop <- "stop" stop-if-true
            w191 = 2
            w193 = string[] ["pmt voltage", "lamp voltage", "lamp int", "internal temp", "react temp", "pres", "flow", "flags"]
            # ">>Monitor command enter as a pair>>"
            # ">>Main commands>>"
            # ">>Monitor Command>>"
            n188 = Array Size(array=w193) -> (size(s)=w194:i32)
            n189 = Divide(x=w194, y=w191) -> (x/y=w192:dbl)
            n190 = for {
              N: w192 -> [_]
              tunnel: w201 -> [w209]
              tunnel: w200 -> [w208]
              tunnel: [w216] -> w190
              shift-right: [w214] -> w196
              shift-left: w197 -> [w215]
              tunnel: [w213] -> w199
              tunnel: w198 -> [w212]
              tunnel: w193 -> [w205]
              tunnel: "so2" -> [w210]
              tunnel: w191 -> [w206]
              tunnel: w188 -> [w202]
              i -> [w207]
              # "FOR Loop runs according\nto the number of monitor commands"
              # "Assemble command:\nso2\npmt voltage\nlamp voltage\n\netc\netc\n\nso2\nflow\nflags"
              n191 = Multiply(x=w206, y=w207) -> (x*y=w203:i32)
              n192 = Array Subset(array=w205, index=w203, length=w206) -> (w204:string[])
              n193 = Build Array (concatenate)(w210, w204) -> (w211:string[])
              "Data In Array" <- w211
              n194 = while {
                tunnel: [w228] -> w216
                tunnel: w211 -> [w226]
                tunnel: [w224] -> w213
                tunnel: w212 -> [w223]
                tunnel: w208 -> [w222]
                tunnel: w209 -> [w221]
                tunnel: w203 -> [w220]
                shift-right: [w225] -> w214
                shift-left: w215 -> [w227]
                tunnel: w202 -> [w217]
                stop <- TRUE stop-if-true
                # "Receive data is organised as:\nDate Time so2 DATA -1\nDate Time pmt voltage DATA 0\nDate Time lamp voltage DATA 1\nDate Time so2 DATA -1\nDate Time lamp int DATA 2\nDate Time internal temp DATA 3\nDate Time so2 DATA -1\nDate Time react temp DATA 4\nDate Time pres DATA 5\nDate Time so2 DATA -1\nDate Time flow DATA 6\nDate Time flags DATA 7\n\nDate Time Read Error -2"
                n195 = for {
                  tunnel: w222 -> [w245]
                  tunnel: [w246] -> w228
                  tunnel: w226 -> [w243] mode=indexing
                  tunnel: [w247] -> w224
                  tunnel: w223 -> [w253]
                  tunnel: w221 -> [w248]
                  tunnel: w220 -> [w242]
                  shift-right: [w257] -> w225
                  shift-left: w227 -> [w258]
                  tunnel: w217 -> [w231]
                  i -> [w235]
                  # "Must insert a wait in order to acquire SO2 43c data"
                  # "Acquire every 330msec for 3 times\nto make 1 second"
                  # "SO2 Acquisition Loop"
                  n196 = call "Wait"("Count(mSec)"=w231) -> ()  [unwired: 1 out]
                  n197 = Concatenate Strings("ID", w243, "\r") -> (w241:string)
                  "Command In" <- w241
                  n198 = call "SO2 Serial Packet Write.vi"("VISA resource name In"=w248, "Data in"=w241, "error in (no error)"=w245) -> ("VISA resource name Out"=w250:refnum<visa-resource-name>, "error out"=w249:errorcluster)  [unwired: 11 in]
                  n199 = call "SO2 Serial Packet Read.vi"("VISA resource In"=w250, "error in"=w249) -> ("VISA resource Out"=w247:refnum<visa-resource-name>, "Data Out"=w238:string, "error out"=w246:errorcluster)  [unwired: 11 in]
                  "RAW DATA" <- w238
                  n200 = Equal?(x=w238, y="Read Error") -> (x = y?=w236:bool)
                  n201 = Get Date/Time In Seconds() -> (seconds since 1Jan1904=w230:timestamp)
                  n202 = case shown="False" w236 {
                    tunnel: [w261 "-2"] -> w251
                    tunnel: w235 -> [w260 _]
                    tunnel: w242 -> [w259 _]
                    frame False {
                      n203 = case shown="0" w260 {
                        tunnel: ["-1" w265 w267] -> w261
                        tunnel: w259 -> [_ w263 w266]
                        frame 0 {
                          # "Make internal flag\n-1 represent so2 data"
                        }
                        frame 2 {
                          # "Make internal flag"
                          n204 = Increment(x=w263) -> (x+1=w264:i32)
                          n205 = Number To Decimal String(number=w264) -> (decimal integer string=w265:string)  [unwired: 1 in]
                        }
                        frame 1, Default {
                          # "Make internal flag"
                          n206 = Number To Decimal String(number=w266) -> (decimal integer string=w267:string)  [unwired: 1 in]
                        }
                      }
                    }
                    frame True {
                    }
                  }
                  n207 = Increment(x=w258) -> (x+1=w254:i32)
                  n208 = Unbundle(w246) -> ("status"=w255:bool)  [unwired: 2 out]
                  n209 = call <vilib>:"Trim Whitespace.vi"("string"=w238) -> ("trimmed string"=w252:string)  [unwired: 1 in]
                  n210 = To Unsigned Long Integer(number=w230) -> (unsigned 32bit integer=w234:u32)
                  n211 = Subtract(x=w234, y=u32 2082844800) -> (x-y=w229:u32)
                  n212 = Select(t=w254, s=w255, f=w258) -> (s? t:f=w257:i32)
                  n213 = call <vilib>:"Space Constant.vi"() -> ("String"=w239:string)
                  n214 = Number To Decimal String(number=w229) -> (decimal integer string=w232:string)  [unwired: 1 in]
                  n215 = Build Array(w232, w239, w252, w239, w251) -> (w240:string[])
                  n216 = Enqueue Element(queue=w253, element=w240) -> ()  [unwired: 2 in, 3 out]
                }
                "Number of Send & Read Error\nfrom Acquire Loop" <- w225
                n217 = call "Wait Until Next Multiple"("Count(mSec)"=u32 1000) -> ()  [unwired: 1 out]
              }
            }
          }
          n218 = node-c288() -> ()  [unwired: 1 in, 1 out]
        }
      }
      n219 = node-c288() -> (w64:T3)  [unwired: 4 in]
      n220 = node-c288() -> (w66:T3)  [unwired: 4 in]
      n221 = timed-loop {
        tunnel: w70 -> [w282]
        timing: w64 -> [_]
        timing-out: [_] -> w63
        stop <- w283 stop-if-true
        # "10 minutes SO2 Average calculated every second"
        n222 = node-c288() -> ()  [unwired: 1 in, 1 out]
        n223 = Get Queue Status(queue=w282, return elements? (F)=TRUE) -> (elements=w273:dbl[])  [unwired: 1 in, 7 out]
        n224 = for {
          tunnel: w273 -> [w286] mode=indexing
          tunnel: [w290] -> w279
          shift-right: [w289] -> w277
          shift-left: i64 0 -> [w288]
          i -> [w290]
          n225 = To Quad Integer(1:w286) -> (0:w287:i64)
          n226 = Add(x=w288, y=w287) -> (x+y=w289:i64)
        }
        n227 = Increment(x=w279) -> (x+1=w274:i32)
        "q_size" <- w274
        n228 = To Double Precision Float(number=w277) -> (double precision float=w275:dbl)
        n229 = To Double Precision Float(number=w274) -> (double precision float=w276:dbl)
        n230 = Divide(x=w275, y=w276) -> (x/y=→"10min_so2_avg":dbl)
        n231 = local read "stop"() -> (w283:bool)
        n232 = node-c288() -> ()  [unwired: 1 in, 1 out]
      }
      n233 = timed-loop {
        tunnel: w69 -> [w302]
        timing: w66 -> [_]
        timing-out: [_] -> w65
        stop <- w303 stop-if-true
        # "8 hours SO2 Average calculated every second"
        n234 = node-c288() -> ()  [unwired: 1 in, 1 out]
        n235 = Get Queue Status(queue=w302, return elements? (F)=TRUE) -> (elements=w299:dbl[])  [unwired: 1 in, 7 out]
        n236 = for {
          tunnel: w299 -> [w306] mode=indexing
          tunnel: [w310] -> w298
          shift-right: [w309] -> w296
          shift-left: i64 0 -> [w308]
          i -> [w310]
          n237 = To Quad Integer(1:w306) -> (0:w307:i64)
          n238 = Add(x=w308, y=w307) -> (x+y=w309:i64)
        }
        n239 = Increment(x=w298) -> (x+1=w293:i32)
        "q_size 2" <- w293
        n240 = To Double Precision Float(number=w296) -> (double precision float=w294:dbl)
        n241 = To Double Precision Float(number=w293) -> (double precision float=w295:dbl)
        n242 = Divide(x=w294, y=w295) -> (x/y=→"8hr_so2_avg 2":dbl)
        n243 = local read "stop"() -> (w303:bool)
        n244 = node-c288() -> ()  [unwired: 1 in, 1 out]
      }
      n245 = node-c288(w65) -> ()  [unwired: 1 out]
      n246 = node-c288(w63) -> ()  [unwired: 1 out]
      n247 = node-c288(w89) -> ()  [unwired: 1 out]
      n248 = while {
        stop <- FALSE stop-if-true
        n249 = node-c288() -> (w94:T3)  [unwired: 4 in]
        n250 = Create Network Stream Reader Endpoint(7:10 ("reader buffer size"), 9:T2 {"Message"="", "Message Data"=variant} ("Message Cluster"), 11:"/command/reader/SO2" ("reader url")) -> (0:w100:errorcluster, 3:w101:refnum<k21>)  [unwired: 4 in]
        n251 = timed-loop "Host->Target Command Reader" {
          shift-right: [w111] -> w98
          shift-left: w100 -> [w114]
          shift-right: [w112] -> w97
          shift-left: w101 -> [w113]
          tunnel: [TRUE] -> _
          timing: w94 -> [_]
          timing-out: [_] -> w93
          stop <- w105 stop-if-true
          # "Receive Commands from Host VI"
          n252 = node-c288() -> ()  [unwired: 1 in, 1 out]
          n253 = shared-variable-read(w113, w114) -> (w112:refnum<k21>, w107:errorcluster, w109:bool, w110:T2)  [unwired: 1 in]
          n254 = Or(x=w109, y=w107) -> (x .or. y?=w108:bool)
          n255 = case shown="False" w108 {
            selector: w108 -> [_ w170]
            tunnel: w107 -> [w122 w171]
            tunnel: [w121 w171] -> w111
            tunnel: w110 -> [w119 _]
            tunnel: [w120 w170] -> w105
            frame False {
              n256 = Unbundle By Name(w119) -> ("Message"=w118:string, "Message Data"=w117:variant)
              n257 = case shown="\"Slope\"" w118 {
                tunnel: w122 -> [w124 w129 w134 w139 w144 w148 w153 w158 w163 w169]
                tunnel: [w124 w126 w132 w137 w143 w146 w151 w156 w161 w166] -> w121
                tunnel: w117 -> [_ w128 w133 w138 w142 w149 w154 w159 w164 w168]
                tunnel: [TRUE _ _ _ _ _ _ _ _ _] -> w120
                frame "Stop", Default {
                }
                frame "Flight Number" {
                  n258 = Variant To Data(error in=w129, type="", Variant=w128) -> (data=→"Flight Number":string, error out=w126:errorcluster)
                }
                frame "10mins STEL Limit" {
                  n259 = Variant To Data(error in=w134, type=0, Variant=w133) -> (data=→"10mins_STEL_limit":i32, error out=w132:errorcluster)
                }
                frame "8hr TWA Limit" {
                  n260 = Variant To Data(error in=w139, type=0, Variant=w138) -> (data=→"8hr_TWA_limit":i32, error out=w137:errorcluster)
                }
                frame "Simulate Conc" {
                  n261 = Variant To Data(error in=w144, type=FALSE, Variant=w142) -> (data=→"Simulate\nconc":bool, error out=w143:errorcluster)
                }
                frame "Simulate STEL Conc" {
                  n262 = Variant To Data(error in=w148, type=0.0, Variant=w149) -> (data=→"Simulate STEL Conc":dbl, error out=w146:errorcluster)
                }
                frame "Simulate TWA Conc" {
                  n263 = Variant To Data(error in=w153, type=0.0, Variant=w154) -> (data=→"Simulate TWA Conc":dbl, error out=w151:errorcluster)
                }
                frame "Offset" {
                  n264 = Variant To Data(error in=w158, type=0.0, Variant=w159) -> (data=→"Offset":dbl, error out=w156:errorcluster)
                }
                frame "Slope" {
                  n265 = Variant To Data(error in=w163, type=0.0, Variant=w164) -> (data=→"Slope":dbl, error out=w161:errorcluster)
                }
                frame "Stop File Write" {
                  n266 = Variant To Data(error in=w169, type=FALSE, Variant=w168) -> (data=→"Stop File Write":bool, error out=w166:errorcluster)
                }
              }
            }
            frame True {
            }
          }
          n267 = node-c288() -> ()  [unwired: 1 in, 1 out]
        }
        n268 = node-c288(w93) -> ()  [unwired: 1 out]
        n269 = Destroy Stream Endpoint(8:w98, 11:w97) -> (0:→"error out 4":errorcluster)
        n270 = Wait (ms)(milliseconds to wait=u32 1000) -> ()  [unwired: 1 out]
      }
      n271 = while {
        tunnel: w77 -> [w355]
        stop <- w356 stop-if-true
        # "UDP Broadcast loop"
        # "Broadcast SO2 UDP Packet"
        n272 = node-c288() -> (w358:T3)  [unwired: 4 in]
        n273 = String To IP(1:"239.1.4.6" ("name")) -> (0:w360:u32)
        n274 = call-poly <vilib>:"UDP Multicast Open.vi"("time-to-live (1)"=u16 5, "port"=u16 10001) -> ("error out"=w368:errorcluster, "connection ID"=w369:refnum<k16>)  [unwired: 8 in]
        n275 = timed-loop {
          tunnel: w369 -> [w389]
          tunnel: w368 -> [w388]
          tunnel: [w375] -> w364
          shift-right: [w378] -> _
          shift-left: FALSE -> [w381]
          tunnel: [w373] -> w362
          tunnel: w360 -> [w377]
          tunnel: u16 50001 ("port or service name") -> [w376]
          timing: w358 -> [_]
          timing-out: [_] -> w357
          tunnel: [w371] -> w356
          tunnel: w355 -> [w370]
          stop <- w372 stop-if-true
          n276 = node-c288() -> ()  [unwired: 1 in, 1 out]
          n277 = local read "Flight Number"() -> (w384:string)
          n278 = Select(t=FALSE, s=w381, f=TRUE) -> (s? t:f=w378:bool)
          "UDP packet \nstatus" <- w378
          n279 = feedback-in #2(w384) -> ()
          n280 = feedback #2() -> (w383:string)  [unwired: 1 in]
          n281 = Not Equal?(x=w384, y=w383) -> (x != y?=w382:bool)
          n282 = flat-sequence {
            tunnel: w377 -> [w397]
            tunnel: w388 -> [w398]
            tunnel: w389 -> [w399]
            tunnel: [w399] -> w387
            tunnel: [w398] -> w386
            tunnel: [w397] -> w385
            tunnel: w382 -> [w396]
            tunnel: w376 -> [w409]
            tunnel: w387 -> [w408]
            tunnel: w386 -> [w407]
            tunnel: w385 -> [w406]
            tunnel: [w405] -> w375
            tunnel: [w404] -> w373
            tunnel: w370 -> [w403]
            frame #0 {
              n283 = feedback #3(u32 0) -> (w393:u32)
              n284 = case shown="True" w396 {
                tunnel: w393 -> [w400 _]
                tunnel: [w400 u32 0] -> w392
                frame False {
                }
                frame True {
                }
              }
              "UDP_Pack_num" <- w392
              n285 = Increment(x=w392) -> (x+1=w394:u32)
              n286 = feedback-in #3(w394) -> ()
            }
            frame #1 {
              n287 = Dequeue Element(queue=w403) -> (element=w402:string)  [unwired: 2 in, 3 out]
              n288 = UDP Write(address=w406, port or service name=w409, connection ID=w408, data in=w402, 8:w407) -> (error out=w404:errorcluster, 3:w405:refnum<k16>)  [unwired: 1 in]
            }
          }
          n289 = local read "stop"() -> (w371:bool)
          n290 = Unbundle(w373) -> ("status"=w374:bool)  [unwired: 2 out]
          n291 = node-c288() -> ()  [unwired: 1 in, 1 out]
          n292 = Compound Arithmetic op=OR(w374, w371) -> (w372:bool)
        }
        n293 = node-c288(w357) -> ()  [unwired: 1 out]
        n294 = UDP Close(connection ID=w364, 8:w362) -> (error out=→"UDP_Out_Error":errorcluster)  [unwired: 1 out]
      }
      n295 = while {
        tunnel: w74 -> [w315]
        tunnel: w75 -> [w314]
        stop <- w318 stop-if-true
        # "TCP Loop writing to SEPTIC Tank"
        n296 = TCP Open Connection(address="192.168.101.108", remote port or service name=u16 3502) -> (connection ID=w321:refnum<k5>, error out=w316:errorcluster)  [unwired: 3 in]
        n297 = case shown="No Error" w316 {
          selector: w316 -> [w326 w353]
          tunnel: w321 -> [w331 w354]
          tunnel: [w330 w354] -> w320
          tunnel: [w329 w353] -> w319
          tunnel: [w328 w352] -> w318
          tunnel: w314 -> [w325 _]
          tunnel: w315 -> [w324 _]
          frame No Error {
            n298 = node-c288() -> (w333:T3)  [unwired: 4 in]
            n299 = timed-loop {
              tunnel: w331 -> [w347]
              tunnel: w326 -> [w346]
              tunnel: [w345] -> w330
              tunnel: [w344] -> w329
              tunnel: [w334] -> w328
              shift-right: [w338] -> _
              shift-left: FALSE -> [w341]
              timing: w333 -> [_]
              timing-out: [_] -> w332
              tunnel: w325 -> [w337]
              tunnel: w324 -> [w336]
              stop <- w342 stop-if-true
              n300 = node-c288() -> ()  [unwired: 1 in, 1 out]
              n301 = Dequeue Element(queue=w337, error in (no error)=w336) -> (element=w335:string)  [unwired: 1 in, 3 out]
              n302 = Select(t=FALSE, s=w341, f=TRUE) -> (s? t:f=w338:bool)
              "TCP packet\nSend to SEPTIC" <- w338
              n303 = TCP Write(connection ID=w347, data in=w335, error in (no error)=w346) -> (connection ID out=w345:refnum<k5>, error out=w344:errorcluster)  [unwired: 1 in, 1 out]
              n304 = local read "stop"() -> (w334:bool)
              n305 = Unbundle(w344) -> ("status"=w343:bool)  [unwired: 2 out]
              n306 = node-c288() -> ()  [unwired: 1 in, 1 out]
              n307 = Compound Arithmetic op=OR(w343, w334) -> (w342:bool)
            }
            n308 = node-c288(w332) -> ()  [unwired: 1 out]
          }
          frame Error {
            n309 = local read "stop"() -> (w352:bool)
          }
        }
        n310 = TCP Close Connection(connection ID=w320, error in (no error)=w319) -> (error out=→"SEPTIC TCP Error Out":errorcluster)  [unwired: 1 in, 1 out]
        n311 = Wait (ms)(milliseconds to wait=u32 1000) -> ()  [unwired: 1 out]
      }
      n312 = while {
        tunnel: w81 -> [w414]
        tunnel: w80 -> [w413]
        stop <- w417 stop-if-true
        # "TCP Loop writing to FISH Tank"
        n313 = TCP Open Connection(address="192.168.101.110", remote port or service name=u16 3502) -> (connection ID=w420:refnum<k5>, error out=w415:errorcluster)  [unwired: 3 in]
        n314 = case shown="No Error" w415 {
          selector: w415 -> [w425 w452]
          tunnel: w420 -> [w430 w453]
          tunnel: [w429 w453] -> w419
          tunnel: [w428 w452] -> w418
          tunnel: [w427 w451] -> w417
          tunnel: w414 -> [w424 _]
          tunnel: w413 -> [w423 _]
          frame No Error {
            n315 = node-c288() -> (w432:T3)  [unwired: 4 in]
            n316 = timed-loop {
              tunnel: w430 -> [w446]
              tunnel: w425 -> [w445]
              tunnel: [w444] -> w429
              tunnel: [w443] -> w428
              tunnel: [w440] -> w427
              shift-right: [w436] -> _
              shift-left: FALSE -> [w439]
              timing: w432 -> [_]
              timing-out: [_] -> w431
              tunnel: w424 -> [w435]
              tunnel: w423 -> [w434]
              stop <- w441 stop-if-true
              n317 = node-c288() -> ()  [unwired: 1 in, 1 out]
              n318 = Dequeue Element(queue=w435, error in (no error)=w434) -> (element=w433:string)  [unwired: 1 in, 3 out]
              n319 = Select(t=FALSE, s=w439, f=TRUE) -> (s? t:f=w436:bool)
              "TCP packet\nSend to FISH" <- w436
              n320 = TCP Write(connection ID=w446, data in=w433, error in (no error)=w445) -> (connection ID out=w444:refnum<k5>, error out=w443:errorcluster)  [unwired: 1 in, 1 out]
              n321 = local read "stop"() -> (w440:bool)
              n322 = Unbundle(w443) -> ("status"=w442:bool)  [unwired: 2 out]
              n323 = node-c288() -> ()  [unwired: 1 in, 1 out]
              n324 = Compound Arithmetic op=OR(w442, w440) -> (w441:bool)
            }
            n325 = node-c288(w431) -> ()  [unwired: 1 out]
          }
          frame Error {
            n326 = local read "stop"() -> (w451:bool)
          }
        }
        n327 = TCP Close Connection(connection ID=w419, error in (no error)=w418) -> (error out=→"FISH TCP Error Out":errorcluster)  [unwired: 1 in, 1 out]
        n328 = Wait (ms)(milliseconds to wait=u32 1000) -> ()  [unwired: 1 out]
      }
      n329 = node-c288(w59) -> ()  [unwired: 1 out]
    }
    frame Error {
    }
  }
  n330 = VISA Close(VISA resource name=w36, error in (no error)=w35) -> (error out=→"Serial Visa Error":errorcluster)
